vi "Set IPS PSU Targets.vi"(8 "error in (no error)":errorcluster, 9 "Target Field Rate (T/min)":dbl format="%#.2f", 10 "Target Field (T)":dbl format="%#.2f", 11 "Instrument.OxfordVRM in":refnum<class "Instrument.OxfordVRM.lvclass">) -> (0 "error out":errorcluster, 2 "Response":string, 3 "Instrument.OxfordVRM out":refnum<class "Instrument.OxfordVRM.lvclass">)   [LabVIEW 2016, in "Instrument.OxfordVRM.lvclass"]
uses:
  Instrument.OxfordVRM.lvclass
  Instrument.OxfordVRM.lvclass/Instrument.OxfordVRM.ctl
  <instrlib>/Mercury iXX/Public/Libraries/Magnet/Open/Open Magnet Device.vi
  <instrlib>/Mercury iXX/Public/Libraries/Magnet/Signals/Set/Target Field Rate (Set).vi
  <instrlib>/Mercury iXX/Public/Libraries/Magnet/Signals/Set/Target Field (Set).vi
  <instrlib>/Mercury iXX/Public/Libraries/Magnet/Signals/Read/Target Field Rate (Read).vi
  <instrlib>/Mercury iXX/Public/Libraries/Magnet/Signals/Read/Target Field (Read).vi
  <instrlib>/Mercury iXX/Mercury iXX.lvlib
  <instrlib>/Mercury iXX/Public/Libraries/Magnet.lvlib
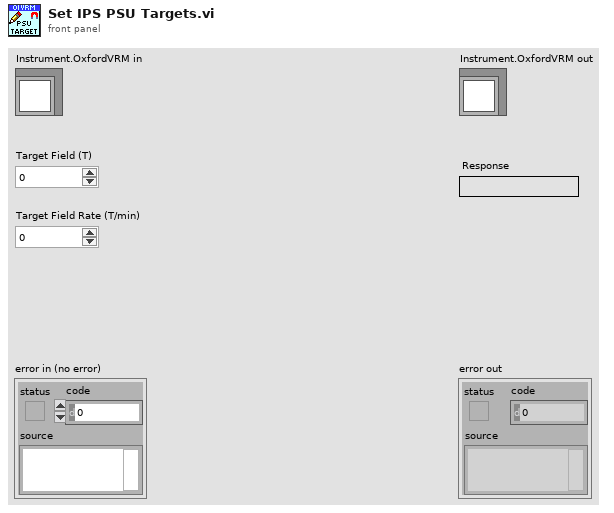
[diagram p1: front panel]
types:
  T1 = typedef "Mercury iXX.lvlib/Mercury Reference.ctl" = cluster{"Comms":refnum<visa-resource-name>, "Device ID":string[], "Comms Layer":T2, "Command":string, "Query reference":T3}
  T2 = typedef "Mercury iXX.lvlib/Comms Transport Layer.ctl" = enum16{"Ethernet TCP/IP", "USB", "ISOBus - RS-232", "GPIB"}
  T3 = typedef "Mercury iXX.lvlib/Query Dynamic Reference.ctl" = refnum<vi>
  T4 = typedef "Mercury iXX.lvlib/Response String.ctl" = string
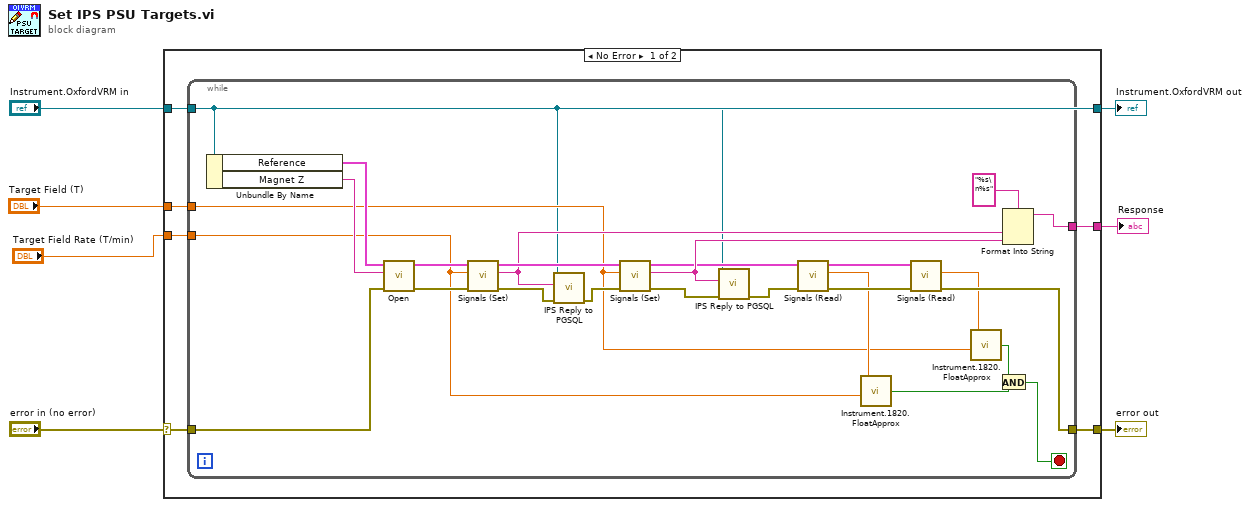
[diagram p0: block diagram]
diagram:
  n1 = case shown="No Error" "error in (no error)" {
    selector: "error in (no error)" -> [w12 w41]
    tunnel: [w8 w41] -> w6
    tunnel: [w13 w40] -> w4
    tunnel: "Instrument.OxfordVRM in" -> [w13 w40]
    tunnel: [w9 _] -> w3
    tunnel: "Target Field (T)" -> [w11 _]
    tunnel: "Target Field Rate (T/min)" -> [w10 _]
    frame No Error {
      n2 = while {
        tunnel: w13 -> [w14]
        tunnel: w12 -> [w38]
        tunnel: w11 -> [w15]
        tunnel: w10 -> [w16]
        tunnel: [w28] -> w9
        tunnel: [w22] -> w8
        stop <- w17 stop-if-true
        n3 = Unbundle By Name(w14) -> ("Reference"=w39:T1, "Magnet Z"=w23:string)
        n4 = call-poly <instrlib>:"Open.vi"("error in (no error)"=w38, "Device Identifier"=w23, "Mercury Reference In"=w39) -> ("error out"=w32:errorcluster, "Mercury Reference Out"=w33:T1)  [unwired: 7 out]
        n5 = call-poly <instrlib>:"Signals (Set).vi"("error in"=w32, "Target Field Rate"=w16, "Mercury Reference In"=w33) -> ("error out"=w36:errorcluster, "Response"=w29:T4, "Mercury Reference Out"=w34:T1)  [unwired: 2 in, 4 out]
        n6 = call "IPS Reply to PGSQL.vi"("error in (no error)"=w36, "Response"=w29, "Instrument.1820 in"=w14) -> ("error out"=w35:errorcluster)  [unwired: 7 in, 1 out]
        n7 = call-poly <instrlib>:"Signals (Set).vi"("error in"=w35, "Target Field"=w15, "Mercury Reference In"=w34) -> ("error out"=w37:errorcluster, "Response"=w30:T4, "Mercury Reference Out"=w26:T1)  [unwired: 2 in, 4 out]
        n8 = call "IPS Reply to PGSQL.vi"("error in (no error)"=w37, "Response"=w30, "Instrument.1820 in"=w14) -> ("error out"=w27:errorcluster)  [unwired: 7 in, 1 out]
        n9 = call-poly <instrlib>:"Signals (Read).vi"("error in"=w27, "Mercury Reference In"=w26) -> ("error out"=w24:errorcluster, "Target Field Rate"=w21:dbl, "Mercury Reference Out"=w25:T1)  [unwired: 5 in, 2 out]
        n10 = call "Instrument.1820.FloatApprox.vi"("y"=w16, "x"=w21) -> ("x ~ y?"=w18:bool)  [unwired: 4 in]
        n11 = call-poly <instrlib>:"Signals (Read).vi"("error in"=w24, "Mercury Reference In"=w25) -> ("error out"=w22:errorcluster, "Target Field"=w20:dbl)  [unwired: 5 in, 3 out]
        n12 = call "Instrument.1820.FloatApprox.vi"("y"=w15, "x"=w20) -> ("x ~ y?"=w19:bool)  [unwired: 4 in]
        n13 = And(x=w19, y=w18) -> (x .and. y?=w17:bool)
        n14 = Format Into String(format string="%s\n%s", w29, w30) -> (resulting string=w28:string)  [unwired: 2 in, 1 out]
      }
    }
    frame Error {
    }
  }
  "error out" <- w6
  "Instrument.OxfordVRM out" <- w4
  "Response" <- w3
